vi "Read-Pressure.vi"(7 "Slave Address (7-bit)":u8 format="%x", 8 "error in (no error)":errorcluster, 9 "T_fine":dbl, 10 "Comp Coeffs":T1 {"dig_H6" format="%0d"; "dig_H5" format="%0d"; "dig_H4" format="%0d"; "dig_H3" format="%0d"; "dig_H2" format="%0d"; "dig_H1" format="%0d"; "dig_P9" format="%0d"; "dig_P8" format="%0d"; "dig_P7" format="%0d"; "dig_P6" format="%0d"; "dig_P5" format="%0d"; "dig_P4" format="%0d"; "dig_P3" format="%0d"; "dig_P2" format="%0d"; "dig_P1" format="%0d"; "dig_T3" format="%0d"; "dig_T2" format="%0d"; "dig_T1" format="%0d"}, 11 "I2C Ref Out in":T2) -> (0 "error out":errorcluster, 1 "T_fine Out":dbl format="%.2f", 2 "Comp Coeffs Out":T1 {"dig_H6" format="%0d"; "dig_H5" format="%0d"; "dig_H4" format="%0d"; "dig_H3" format="%0d"; "dig_H2" format="%0d"; "dig_H1" format="%0d"; "dig_P9" format="%0d"; "dig_P8" format="%0d"; "dig_P7" format="%0d"; "dig_P6" format="%0d"; "dig_P5" format="%0d"; "dig_P4" format="%0d"; "dig_P3" format="%0d"; "dig_P2" format="%0d"; "dig_P1" format="%0d"; "dig_T3" format="%0d"; "dig_T2" format="%0d"; "dig_T1" format="%0d"}, 3 "I2C Ref Out":T2, 4 "ADC RAW PRESSURE":u32, 5 "Bytes Read":u8[](array[numeric]), 6 "p":dbl)   [LabVIEW 2015]
uses:
  <vilib>/myRIO/Instrument Drivers/Onboard IO/I2C/typedefs/I2C Reference.ctl
  <vilib>/myRIO/Common/Instrument Driver Framework/Utilities/typedefs/myRIO Generic Hardware Reference.ctl
  <vilib>/myRIO/Common/Instrument Driver Framework/Utilities/typedefs/Hardware Version Enum.ctl
  <vilib>/myRIO/Common/Instrument Driver Framework/Utilities/typedefs/myRIO v1.0 Reference.ctl
  <vilib>/myRIO/Common/Instrument Driver Framework/Utilities/typedefs/Generic FPGA Reference.ctl
  <vilib>/myRIO/Common/Instrument Driver Framework/myRIO v1.0/I2C/typedefs/I2C Channels Enum.ctl
  <vilib>/myRIO/Instrument Drivers/Onboard IO/I2C/typedefs/I2C Configuration.ctl
  <vilib>/myRIO/Instrument Drivers/Onboard IO/I2C/typedefs/I2C Transfer Rate.ctl
  calib_data.ctl
  <vilib>/Utility/error.llb/Error Cluster From Error Code.vi
  <vilib>/myRIO/Common/Instrument Driver Framework/myRIO v1.0/I2C/vis/myRIO v1.0 Write I2C.vi
  <vilib>/myRIO/Common/Instrument Driver Framework/myRIO v1.0/I2C/vis/myRIO v1.0 Read I2C.vi
  <vilib>/myRIO/Instrument Drivers/Onboard IO/I2C/I2C.lvlib
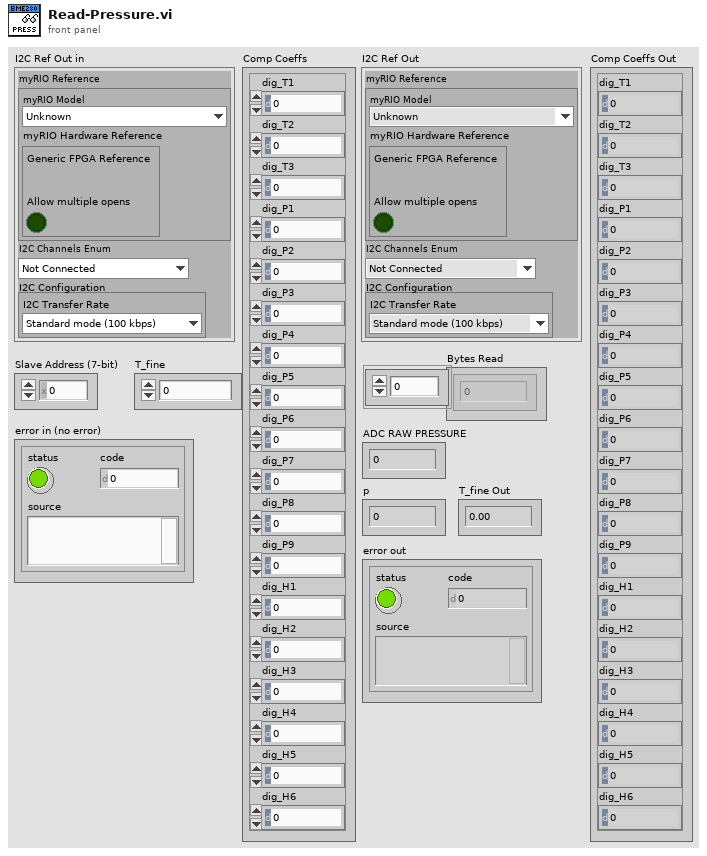
[diagram p1: front panel]
types:
  T1 = typedef "calib_data.ctl" = cluster{"dig_T1":u16, "dig_T2":i16, "dig_T3":i16, "dig_P1":u16, "dig_P2":i16, "dig_P3":i16, "dig_P4":i16, "dig_P5":i16, "dig_P6":i16, "dig_P7":i16, "dig_P8":i16, "dig_P9":i16, "dig_H1":u8, "dig_H2":i16, "dig_H3":u8, "dig_H4":i16, "dig_H5":i16, "dig_H6":i8}
  T2 = typedef "I2C.lvlib/I2C Reference.ctl" = cluster{"myRIO Reference":T3, "I2C Channels Enum":T7, "I2C Configuration":T8}
  T3 = typedef "myRIO Generic Hardware Reference.ctl" = cluster{"myRIO Model":T4, "myRIO Hardware Reference":T5}
  T4 = typedef "Hardware Version Enum.ctl" = enum16{"Unknown", "myRIO-1900", "myRIO-1950", "roboRIO"}
  T5 = typedef "myRIO v1.0 Reference.ctl" = cluster{"Generic FPGA Reference":T6, "Allow multiple opens":bool}
  T6 = typedef "Generic FPGA Reference.ctl" = refnum<k20>
  T7 = typedef "I2C Channels Enum.ctl" = enum16{"Not Connected", "A/I2C", "B/I2C", "I2C/I2C"}
  T8 = typedef "I2C.lvlib/I2C Configuration.ctl" = cluster{"I2C Transfer Rate":T9}
  T9 = typedef "I2C.lvlib/I2C Transfer Rate.ctl" = enum16{"Standard mode (100 kbps)", "Fast mode (400 kbps)"}
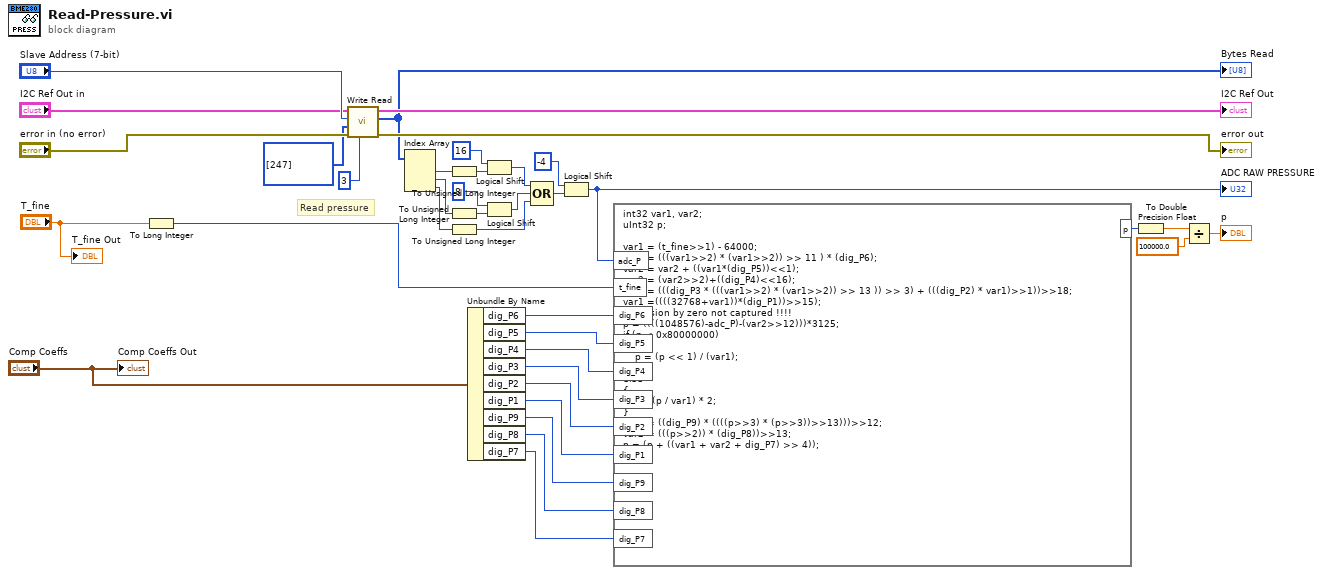
[diagram p0: block diagram]
diagram:
  # "Read pressure"
  n1 = To Long Integer(number="T_fine") -> (32bit integer=w5:i32)
  n2 = call <vilib>:"Write Read.vi"("Byte Count"=u32 3, "error in (no error)"="error in (no error)", "Bytes to Write"=u8[] [247], "Slave Address (7-bit)"="Slave Address (7-bit)", "I2C Ref In"="I2C Ref Out in") -> ("error out"=→"error out":errorcluster, "Bytes Read"=w30:u8[], "I2C Ref Out"=→"I2C Ref Out":T2)  [unwired: 3 in]
  "Bytes Read" <- w30
  n3 = Index Array(array=w30) -> (element #1=w29:u8, element #2=w28:u8, element #3=w27:u8)  [unwired: 3 in]
  n4 = To Unsigned Long Integer(number=w29) -> (unsigned 32bit integer=w21:u32)
  n5 = To Unsigned Long Integer(number=w28) -> (unsigned 32bit integer=w20:u32)
  n6 = To Unsigned Long Integer(number=w27) -> (unsigned 32bit integer=w25:u32)
  n7 = Unbundle By Name("Comp Coeffs") -> ("dig_P6"=w15:i16, "dig_P5"=w14:i16, "dig_P4"=w13:i16, "dig_P3"=w12:i16, "dig_P2"=w11:i16, "dig_P1"=w10:u16, "dig_P9"=w9:i16, "dig_P8"=w8:i16, "dig_P7"=w7:i16)
  n8 = Logical Shift(y=u8 16 ("x"), x=w21) -> (x << y=w26:u32)
  n9 = Logical Shift(y=u8 8 ("x"), x=w20) -> (x << y=w24:u32)
  n10 = Compound Arithmetic op=OR(w26, w24, w25) -> (w19:u32)
  n11 = Logical Shift(y=i16 -4, x=w19) -> (x << y=w16:u32)
  "ADC RAW PRESSURE" <- w16
  n12 = formula code="int32 var1, var2;\nuInt32 p;\n\nvar1 = (t_fine>>1) - 64000;\nvar2 = (((var1>>2) * (var1>>2)) >> 11 ) * (dig_P6);\nvar2 = var2 + ((var1*(dig_P5))<<1);\nvar2 = (var2>>2)+((dig_P4)<<16);\nvar1 = (((dig_P3 * (((var1>>2) * (var1>>2)) >> 13 )) >> 3) + (((dig_P2) * var1)>>1))>>18;\nvar1 =((((32768+var1))*(dig_P1))>>15);\n// Division by zero not captured !!!!\np = ((((1048576)-adc_P)-(var2>>12)))*3125;\nif (p < 0x80000000)\n{\n    p = (p << 1) / (var1);\n}\nelse\n{\n   p = (p / var1) * 2;\n}\nvar1 = ((dig_P9) * ((((p>>3) * (p>>3))>>13)))>>12;\nvar2 = (((p>>2)) * (dig_P8))>>13;\np = (p + ((var1 + var2 + dig_P7) >> 4));"("adc_P"=w16, "dig_P6"=w15, "dig_P5"=w14, "dig_P4"=w13, "dig_P3"=w12, "dig_P2"=w11, "dig_P1"=w10, "dig_P9"=w9, "dig_P8"=w8, "dig_P7"=w7, "t_fine"=w5) -> ("p"=w2:u32)
  n13 = To Double Precision Float(number=w2) -> (double precision float=w1:dbl)
  n14 = Divide(x=w1, y=100000.0) -> (x/y=→"p":dbl)
  "Comp Coeffs Out" <- "Comp Coeffs"
  "T_fine Out" <- "T_fine"
